vi "Simple Reader.vi"(8 "error in (no error)":errorcluster, 11 "MFLI Driver in":refnum<class "MFLI Driver.lvclass">) -> (0 "error out":errorcluster, 2 "Signals":dbl[](array[numeric]), 3 "MFLI Driver out":refnum<class "MFLI Driver.lvclass">)   [LabVIEW 2021, in "MFLI Driver.lvclass"]
uses:
  MFLI Driver.lvclass
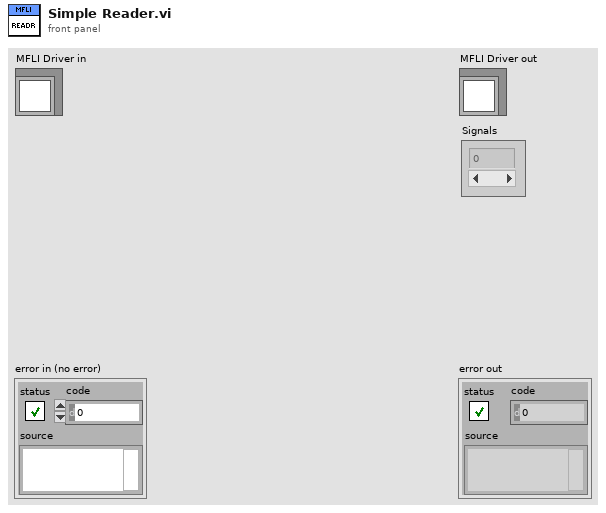
[diagram p1: front panel]
types:
  T1 = typedef "Zurich Instruments LabOne.lvlib/ziTypeHandle.ctl" = cluster{"handleValid":bool, "Conn":u64, "Path Prefix":string, "Handle":u64, "Connected":bool, "Clockbase(s)":dbl}
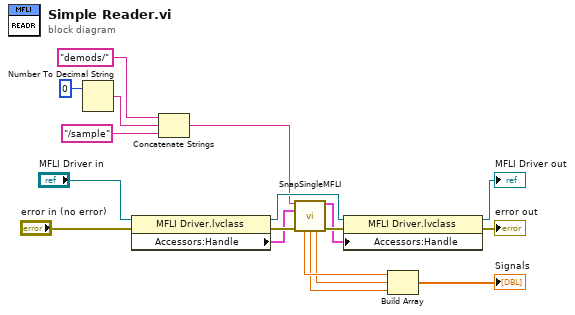
[diagram p0: block diagram]
diagram:
  n1 = Number To Decimal String(number=0) -> (decimal integer string=w11:string)  [unwired: 1 in]
  n2 = property class="MFLI Driver.lvclass"(reference="MFLI Driver in", error in="error in (no error)") -> (reference out=w16:refnum<class "MFLI Driver.lvclass">, error out=w9:errorcluster, "Accessors:Handle"=w7:T1)
  n3 = Concatenate Strings("demods/" ("string"), w11, "/sample" ("string")) -> (w5:string)
  n4 = call "SnapSingleMFLI.vi"("Path"=w5, "Handle in"=w7, "error in (no error)"=w9) -> ("Handle in 2"=w6:T1, "Timestamp(s)"=w4:dbl, "Thera (rad)"=w2:dbl, "R (Vrms)"=w3:dbl, "error out"=w8:errorcluster)  [unwired: 4 in, 4 out]
  n5 = property class="MFLI Driver.lvclass"(reference=w16, error in=w8, "Accessors:Handle"=w6) -> (reference out=→"MFLI Driver out":refnum<class "MFLI Driver.lvclass">, error out=→"error out":errorcluster)
  n6 = Build Array(w4, w3, w2) -> (→"Signals":dbl[])
